vi "Init.vi"(5 "PathControl.lvclass":refnum<class "PathControl.lvclass">, 6 "Environmental classes":refnum<class "Instrument.lvclass">[](array[class]), 7 "XML Handler.lvclass":refnum<class "XML Handler.lvclass">, 8 "error in (no error)":errorcluster, 9 "Instruments to Use":T1(array[cluster]), 10 "Device.lvclass":refnum<class "Device.lvclass">, 11 "LCR-Measurement in":refnum<class "OTP_LCR_Meas.lvclass">) -> (0 "error out":errorcluster, 3 "LCR-Measurement out":refnum<class "OTP_LCR_Meas.lvclass">)   [LabVIEW 2020, in "OTP_LCR_Meas.lvclass"]
doc: "Initializes the measurement.\nThis verifies that the instruments are present and adds them into the class data.\nIs also adds the xml handler into the class data."
uses:
  OTP_LCR_Meas.lvclass
  Devices/Device.lvclass
  Instruments/Instrument.lvclass
  XML Handler/XML Handler.lvclass
  Path Control/PathControl.lvclass
  Controls/Init States.ctl
  Instruments/LCR Meter/LCR Meter.lvclass
  Measurement.lvclass
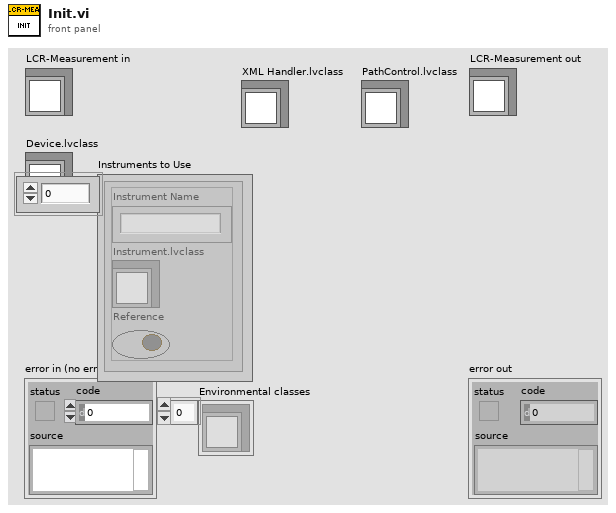
[diagram p1: front panel]
types:
  T1 = cluster{"Instrument Name":string, "Instrument.lvclass":refnum<class "Instrument.lvclass">, "Reference":bool}[]
  T2 = typedef "Measurement.lvclass/Init States.ctl" = enum16{"Verify instruments", "Init Parameters", "Init Instruments", "Add Device", "Init Device", "Create test in XML", "Set path", "Done"}
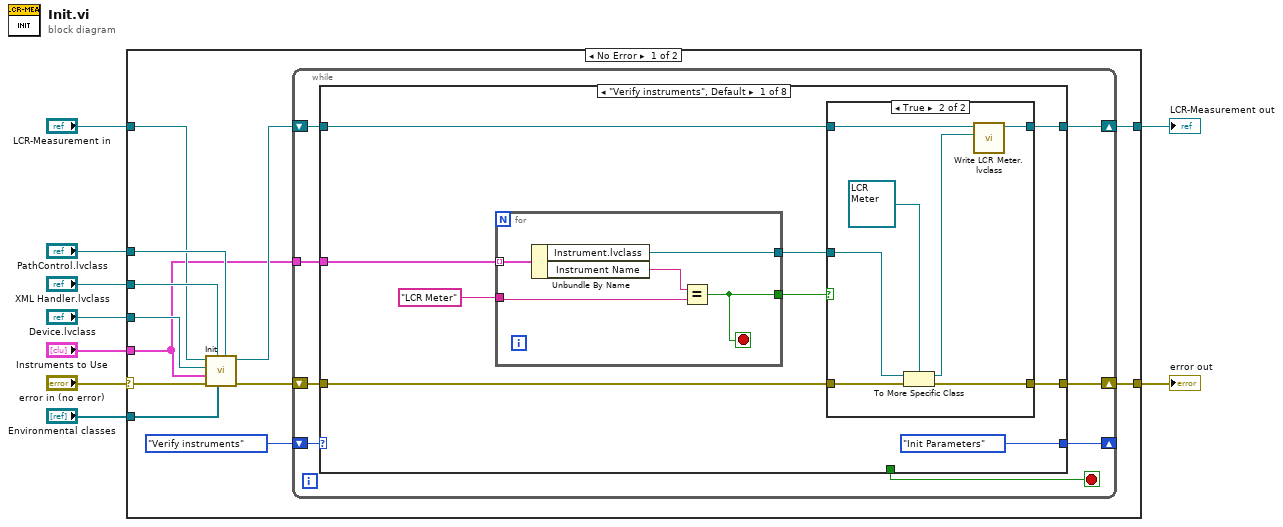
[diagram p0: block diagram]
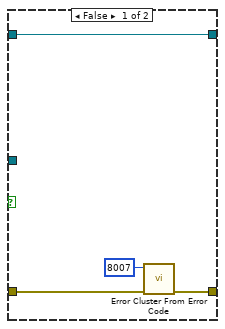
[diagram p2: hidden frame]
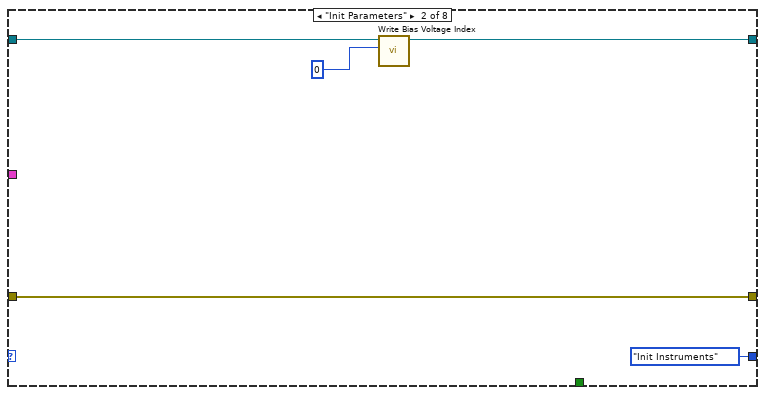
[diagram p3: hidden frame]
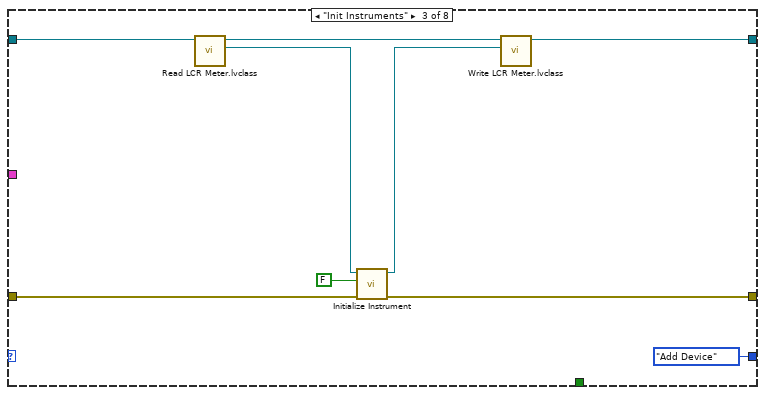
[diagram p4: hidden frame]
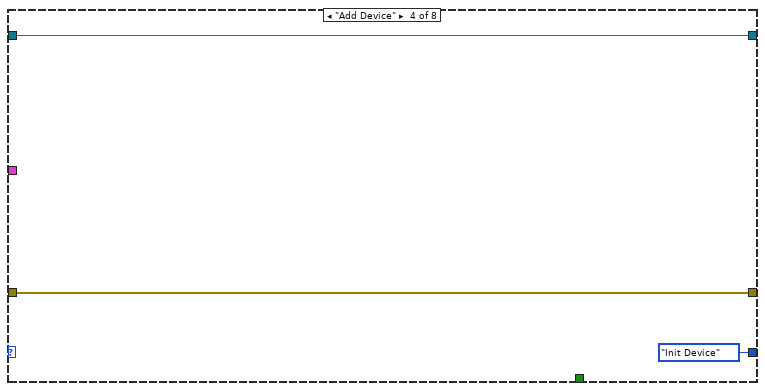
[diagram p5: hidden frame]
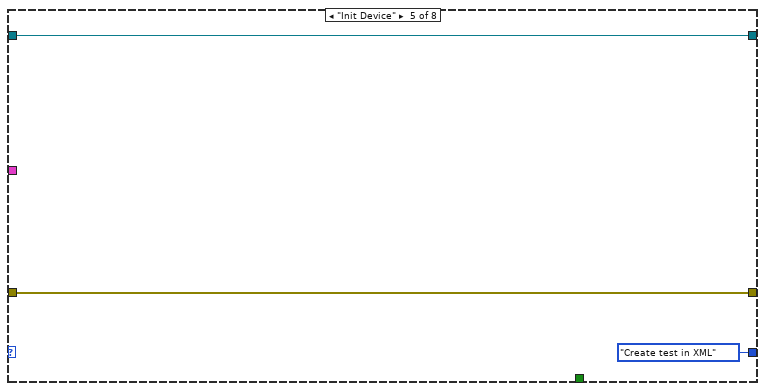
[diagram p6: hidden frame]
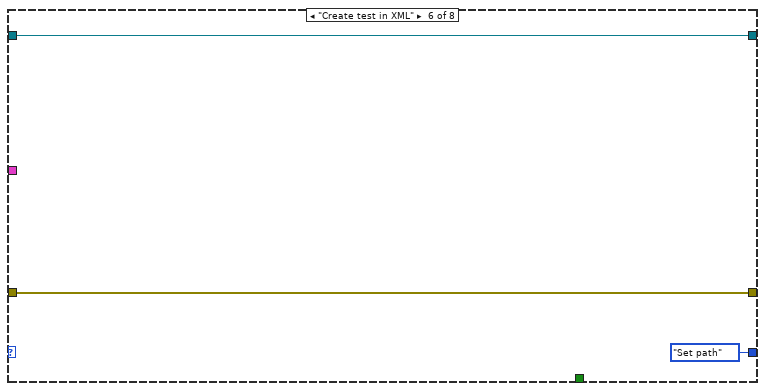
[diagram p7: hidden frame]
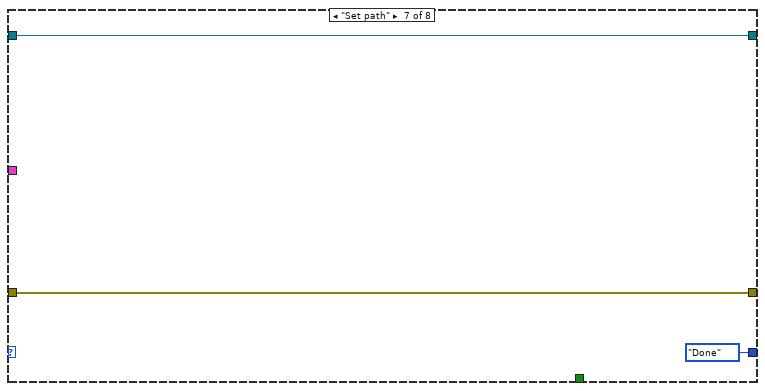
[diagram p8: hidden frame]
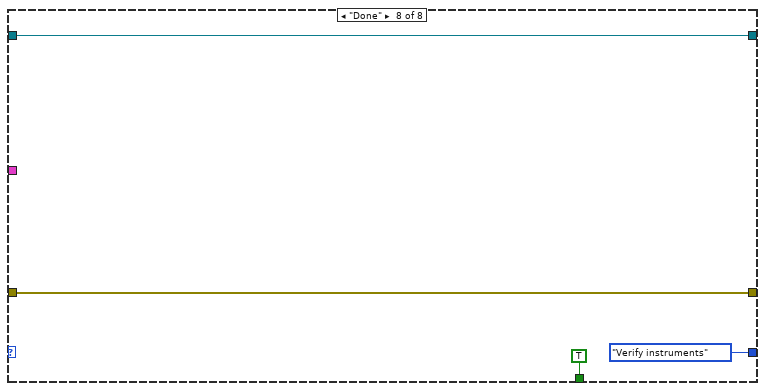
[diagram p9: hidden frame]
diagram:
  n1 = case shown="No Error" "error in (no error)" {
    selector: "error in (no error)" -> [w18 w85]
    tunnel: "PathControl.lvclass" -> [w21 _]
    tunnel: "Environmental classes" -> [w20 _]
    tunnel: "XML Handler.lvclass" -> [w19 _]
    tunnel: "Instruments to Use" -> [w10 _]
    tunnel: "Device.lvclass" -> [w17 _]
    tunnel: "LCR-Measurement in" -> [w16 w86]
    tunnel: [w13 w85] -> w2
    tunnel: [w12 w86] -> w1
    frame No Error {
      n2 = call-parent "Init.vi"("PathControl.lvclass"=w21, "Environmental classes"=w20, "XML Handler.lvclass"=w19, "error in (no error)"=w18, "Instruments to Use"=w10, "Device.lvclass"=w17, "Measurements in"=w16) -> ("error out"=w14:errorcluster, "Measurements out"=w11:refnum<class "OTP_LCR_Meas.lvclass">)  [unwired: 3 in]
      n3 = while {
        shift-right: [w27] -> w13
        shift-left: w14 -> [w28]
        shift-right: [w26] -> w12
        shift-left: w11 -> [w25]
        tunnel: w10 -> [w23]
        shift-right: [w22] -> _
        shift-left: Init_States."Verify instruments" ("Init States") -> [w29]
        stop <- w24 stop-if-true
        n4 = case shown="\"Verify instruments\", Default" w29 {
          tunnel: w28 -> [w32 w59 w67 w71 w74 w77 w80 w84]
          tunnel: [w31 w59 w66 w71 w74 w77 w80 w84] -> w27
          tunnel: [w35 w56 w60 w70 w73 w76 w79 w83] -> w26
          tunnel: w25 -> [w36 w57 w61 w70 w73 w76 w79 w83]
          tunnel: [_ _ _ _ _ _ _ TRUE] -> w24
          tunnel: w23 -> [w38 _ _ _ _ _ _ _]
          tunnel: [Init_States."Init Parameters" ("Init States") Init_States."Init Instruments" ("Init States") Init_States."Add Device" ("Init States") Init_States."Init Device" ("Init States") Init_States."Create test in XML" ("Init States") Init_States."Set path" ("Init States") Init_States."Done" ("Init States") Init_States."Verify instruments" ("Init States")] -> w22
          frame "Verify instruments", Default {
            n5 = for {
              tunnel: w38 -> [w54] mode=indexing
              tunnel: "LCR Meter" -> [w52]
              tunnel: [w51] -> w34
              tunnel: [w50] -> w30
              stop <- w50 stop-if-true
              n6 = Unbundle By Name(w54) -> ("Instrument.lvclass"=w51:refnum<class "Instrument.lvclass">, "Instrument Name"=w53:string)
              n7 = Equal?(x=w53, y=w52) -> (x = y?=w50:bool)
            }
            n8 = case shown="True" w30 {
              tunnel: w36 -> [w40 w49]
              tunnel: [w40 w48] -> w35
              tunnel: w34 -> [_ w47]
              tunnel: w32 -> [w42 w45]
              tunnel: [w41 w44] -> w31
              frame False {
                n9 = call <vilib>:"Error Cluster From Error Code.vi"("error in (no error)"=w42, "error code (0)"=8007) -> ("error out"=w41:errorcluster)  [unwired: 7 in]
              }
              frame True {
                n10 = To More Specific Class(target class=refnum<class "LCR Meter.lvclass"> refnum ("LCR Meter.lvclass"), reference=w47, error in=w45) -> (specific class reference=w46:refnum<class "LCR Meter.lvclass">, error out=w44:errorcluster)
                n11 = call-dynamic "Write LCR Meter.lvclass.vi"("LCR Meter.lvclass"=w46, "LCR-Measurement in"=w49) -> ("LCR-Measurement out"=w48:refnum<class "OTP_LCR_Meas.lvclass">)  [unwired: 9 in]
              }
            }
          }
          frame "Init Parameters" {
            n12 = call-dynamic "Write Bias Voltage Index.vi"("Bias Voltage Index"=0, "LCR-Measurement in"=w57) -> ("LCR-Measurement out"=w56:refnum<class "OTP_LCR_Meas.lvclass">)  [unwired: 9 in]
          }
          frame "Init Instruments" {
            n13 = call-dynamic "Read LCR Meter.lvclass.vi"("LCR-Measurement in"=w61) -> ("LCR Meter.lvclass"=w64:refnum<class "LCR Meter.lvclass">, "LCR-Measurement out"=w62:refnum<class "OTP_LCR_Meas.lvclass">)  [unwired: 9 in]
            n14 = call-dynamic "Initialize Instrument.vi"("error in (no error)"=w67, "Reset"=FALSE, "Instrument in"=w64) -> ("error out"=w66:errorcluster, "Instrument out"=w63:refnum<class "LCR Meter.lvclass">)  [unwired: 7 in]
            n15 = call-dynamic "Write LCR Meter.lvclass.vi"("LCR Meter.lvclass"=w63, "LCR-Measurement in"=w62) -> ("LCR-Measurement out"=w60:refnum<class "OTP_LCR_Meas.lvclass">)  [unwired: 9 in]
          }
          frame "Add Device" {
          }
          frame "Init Device" {
          }
          frame "Create test in XML" {
          }
          frame "Set path" {
          }
          frame "Done" {
          }
        }
      }
    }
    frame Error {
    }
  }
  "error out" <- w2
  "LCR-Measurement out" <- w1
